vi "ISO-TP sequence.vi"(0 "Channel":u16, 1 "MessageBuffer":T2, 2 "No Messages to read":i32, 3 "Response ID":u32, 4 "State":u8 format="%.0x", 5 "error in":errorcluster) -> (13 "MessageBuffer out":T1(array[cluster]), 14 "Channel out":u16, 15 "Answers":T1(array[cluster]), 16 "Boolean 2":bool, 19 "error out":errorcluster)   [LabVIEW 2023, in "PCAN API.lvlib"]
uses:
  PCAN API.lvlib
panel:
  out "Numeric 2":i32
  out "Numeric":i32
  in  "Boolean":bool
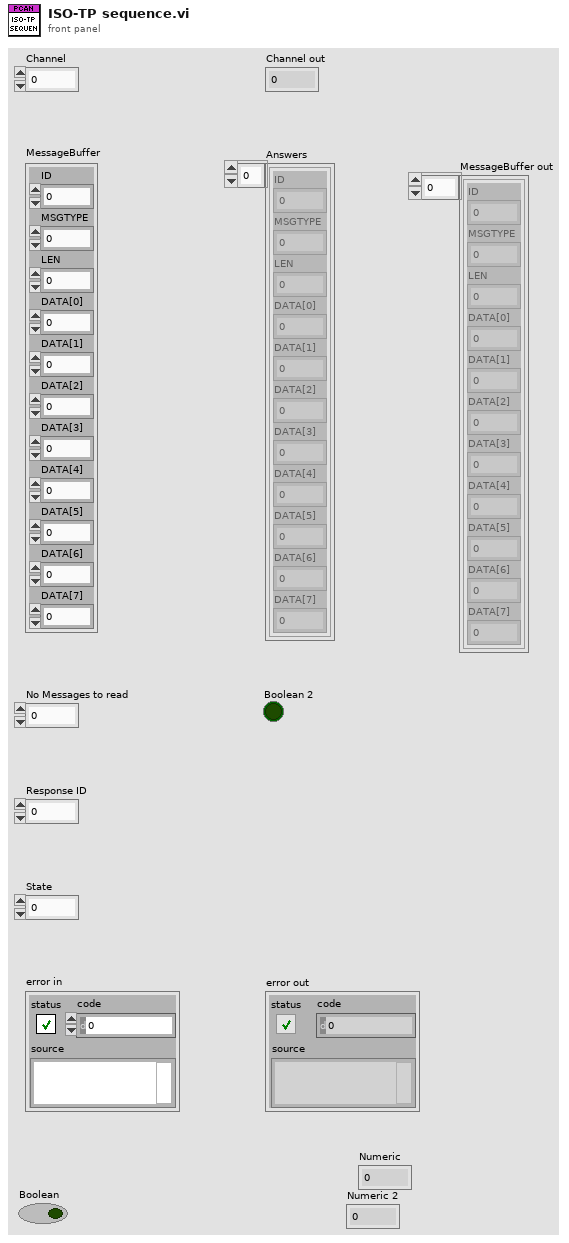
[diagram p1: front panel]
types:
  T1 = cluster{"ID":u32, "MSGTYPE":u8, "LEN":u8, "DATA[0]":u8, "DATA[1]":u8, "DATA[2]":u8, "DATA[3]":u8, "DATA[4]":u8, "DATA[5]":u8, "DATA[6]":u8, "DATA[7]":u8}[]
  T2 = cluster{"ID":u32, "MSGTYPE":u8, "LEN":u8, "DATA[0]":u8, "DATA[1]":u8, "DATA[2]":u8, "DATA[3]":u8, "DATA[4]":u8, "DATA[5]":u8, "DATA[6]":u8, "DATA[7]":u8}
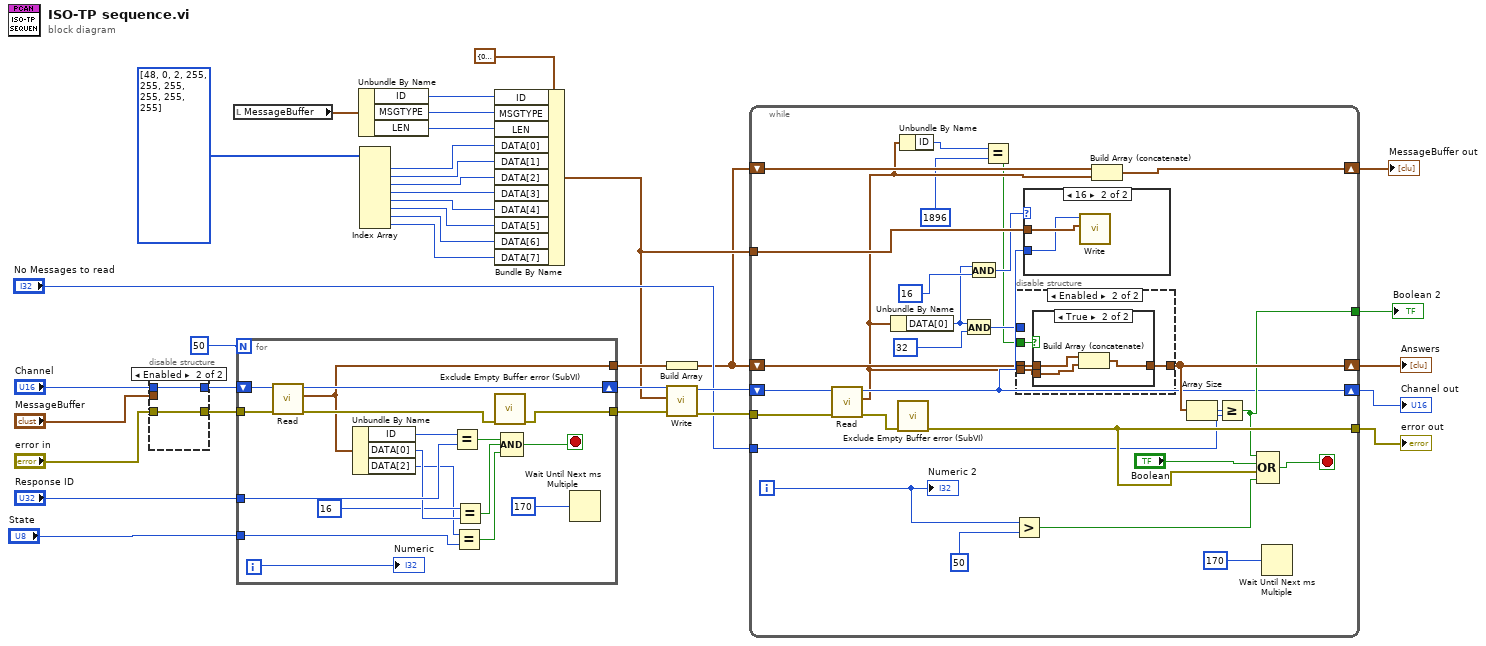
[diagram p0: block diagram]
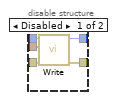
[diagram p2: hidden frame]
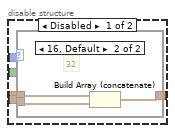
[diagram p3: hidden frame]
diagram:
  n1 = disable-structure shown="Enabled" {
    disable-tunnel: "error in" -> [w40 w41]
    disable-tunnel: [w39 w42] -> w34
    disable-tunnel: [w38 w41] -> w33
    disable-tunnel: "Channel" -> [w37 w42]
    disable-tunnel: "MessageBuffer" -> [w36 _]
    frame Disabled {
      n2 = call "Write.vi"("error in"=w40, "MessageBuffer"=w36, "Channel"=w37) -> ("error out"=w38:errorcluster, "Channel out"=w39:u16)  [unwired: 5 in, 2 out]
    }
    frame Enabled {
    }
  }
  n3 = local read "MessageBuffer"() -> (w23:T2)
  n4 = for {
    N: 50 -> [_]
    tunnel: w33 -> [w59]
    shift-right: [w58] -> w31
    shift-left: w34 -> [w60]
    tunnel: [w52] -> w30
    tunnel: "Response ID" -> [w56]
    tunnel: [w51] -> w27
    tunnel: "State" -> [w47]
    i -> [w49]
    stop <- w43 stop-if-true
    n5 = call "Read.vi"("error in"=w59, "Channel"=w60) -> ("error out"=w53:errorcluster, "MessageBuffer out"=w51:T2, "Channel out"=w58:u16)  [unwired: 6 in, 1 out]
    n6 = Unbundle By Name(w51) -> ("ID"=w57:u32, "DATA[0]"=w55:u8, "DATA[2]"=w48:u8)
    n7 = Equal?(x=w57, y=w56) -> (x = y?=w46:bool)
    n8 = Equal?(x=w48, y=w47) -> (x = y?=w44:bool)
    n9 = Equal?(x=u8 16 ("y"), y=w55) -> (x = y?=w45:bool)
    n10 = call "Exclude Empty Buffer error (SubVI).vi"("error in"=w53) -> ("error out"=w52:errorcluster)  [unwired: 10 in]
    n11 = Compound Arithmetic op=AND(w46, w45, w44) -> (w43:bool)
    n12 = Wait Until Next ms Multiple(millisecond multiple=u32 170) -> ()  [unwired: 1 out]
    "Numeric" <- w49
  }
  n13 = Unbundle By Name(w23) -> ("ID"=w22:u32, "MSGTYPE"=w21:u8, "LEN"=w20:u8)
  n14 = Index Array(array=u8[] [48, 0, 2, 255, 255, 255, 255, 255, 255]) -> (element #1=w14:u8, element #2=w13:u8, element #3=w12:u8, element #4=w11:u8, element #5=w10:u8, element #6=w9:u8, element #7=w8:u8, element #8=w7:u8)  [unwired: 8 in]
  n15 = Bundle By Name(cluster=T2 {"ID"=0, "MSGTYPE"=0, "LEN"=0, "DATA[0]"=0, "DATA[1]"=0, "DATA[2]"=0, "DATA[3]"=0, "DATA[4]"=0, "DATA[5]"=0, "DATA[6]"=0, "DATA[7]"=0} ("MessageBuffer"), "ID"=w22, "MSGTYPE"=w21, "LEN"=w20, "DATA[0]"=w14, "DATA[1]"=w13, "DATA[2]"=w12, "DATA[3]"=w11, "DATA[4]"=w10, "DATA[5]"=w9, "DATA[6]"=w8, "DATA[7]"=w7) -> (w4:T2)
  n16 = Build Array(w27) -> (w1:T1)
  n17 = call "Write.vi"("error in"=w30, "MessageBuffer"=w4, "Channel"=w31) -> ("error out"=w28:errorcluster, "Channel out"=w29:u16)  [unwired: 5 in, 2 out]
  n18 = while {
    tunnel: w28 -> [w87]
    shift-right: [w73] -> w18
    shift-left: w29 -> [w88]
    tunnel: [w83] -> w17
    shift-right: [w81] -> w19
    shift-left: w1 -> [w71]
    tunnel: "No Messages to read" -> [w79]
    tunnel: [w77] -> w5
    tunnel: w4 -> [w74]
    shift-right: [w70] -> w2
    shift-left: w1 -> [w69]
    i -> [w63]
    stop <- w78 stop-if-true
    n19 = call "Read.vi"("error in"=w87, "Channel"=w88) -> ("error out"=w86:errorcluster, "MessageBuffer out"=w68:T2, "Channel out"=w73:u16)  [unwired: 6 in, 1 out]
    n20 = Unbundle By Name(w68) -> ("DATA[0]"=w75:u8)
    n21 = call "Exclude Empty Buffer error (SubVI).vi"("error in"=w86) -> ("error out"=w83:errorcluster)  [unwired: 10 in]
    n22 = Unbundle By Name(w68) -> ("ID"=w67:u32)
    n23 = And(x=w75, y=u8 32) -> (x .and. y?=w65:u8)
    n24 = And(x=w75, y=u8 16) -> (x .and. y?=w72:u8)
    n25 = Equal?(x=w67, y=u32 1896) -> (x = y?=w64:bool)
    n26 = Greater?(x=w63, y=50) -> (0:w61:bool)
    n27 = disable-structure shown="Enabled" {
      disable-tunnel: [w92 w98] -> w81
      disable-tunnel: w71 -> [w91 w99]
      disable-tunnel: w68 -> [w90 w97]
      disable-tunnel: w65 -> [w89 _]
      disable-tunnel: w64 -> [_ w100]
      frame Disabled {
        n28 = case shown="16, Default" w89 {
          tunnel: w91 -> [w93 w96]
          tunnel: w90 -> [_ w95]
          tunnel: [w93 w94] -> w92
          frame 0 {
          }
          frame 16, Default {
            # "32"
            n29 = Build Array (concatenate)(w96, w95) -> (w94:T1)
          }
        }
      }
      frame Enabled {
        n30 = case shown="True" w100 {
          tunnel: w99 -> [w101 w104]
          tunnel: [w101 w103] -> w98
          tunnel: w97 -> [_ w102]
          frame False {
          }
          frame True {
            n31 = Build Array (concatenate)(w104, w102) -> (w103:T1)
          }
        }
      }
    }
    n32 = case shown="16" w72 {
      tunnel: w74 -> [_ w106]
      tunnel: w73 -> [_ w105]
      frame 0, Default {
      }
      frame 16 {
        n33 = call "Write.vi"("MessageBuffer"=w106, "Channel"=w105) -> ()  [unwired: 6 in, 4 out]
      }
    }
    n34 = Build Array (concatenate)(w69, w68) -> (w70:T1)
    n35 = Array Size(array=w81) -> (size(s)=w80:i32)
    n36 = Greater Or Equal?(x=w80, y=w79) -> (x >= y?=w77:bool)
    n37 = Compound Arithmetic op=OR(w77, "Boolean", w83, w61) -> (w78:bool)
    n38 = Wait Until Next ms Multiple(millisecond multiple=u32 170) -> ()  [unwired: 1 out]
    "Numeric 2" <- w63
  }
  "Answers" <- w19
  "Channel out" <- w18
  "error out" <- w17
  "Boolean 2" <- w5
  "MessageBuffer out" <- w2
